vi "_sub_filter_raw_data.vi"(11 "raw data input":u32[](array[numeric])) -> (2 "Filtered raw data index":i32[](array[numeric]), 3 "Filtered raw data":u32[](array[numeric]))   [LabVIEW 2015]
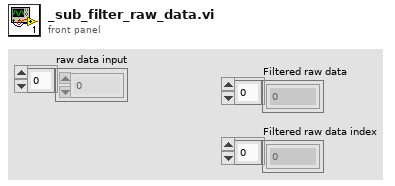
[diagram p1: front panel]
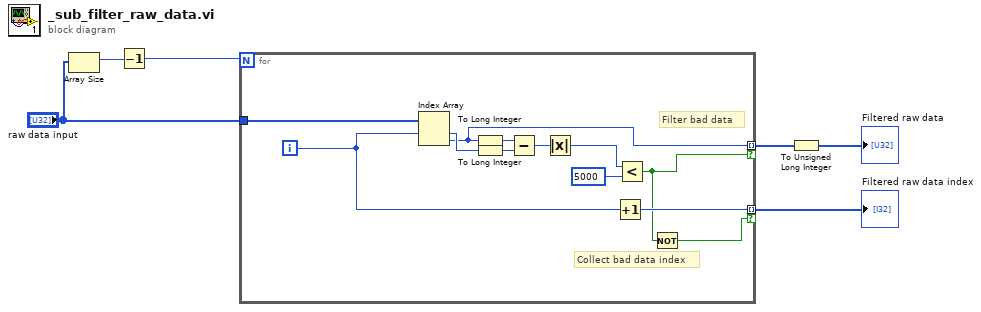
[diagram p0: block diagram]
diagram:
  n1 = Array Size(array="raw data input") -> (size(s)=w2:i32)
  n2 = Decrement(x=w2) -> (x-1=w1:i32)
  n3 = for {
    N: w1 -> [_]
    tunnel: "raw data input" -> [w18]
    tunnel: [w7] -> w6 mode=indexing if=w10
    tunnel: [w11] -> w5 mode=indexing if=w9
    i -> [w12]
    # "Collect bad data index"
    # "Filter bad data"
    n4 = Index Array(array=w18, index #1=w12) -> (element #1=w8:u32, element #2=w7:u32)  [unwired: 1 in]
    n5 = To Long Integer(number=w7) -> (32bit integer=w17:i32)
    n6 = To Long Integer(number=w8) -> (32bit integer=w16:i32)
    n7 = Subtract(x=w17, y=w16) -> (x-y=w15:i32)
    n8 = Absolute Value(x=w15) -> (abs(x)=w14:i32)
    n9 = Increment(x=w12) -> (x+1=w11:i32)
    n10 = Less?(x=w14, y=5000) -> (x < y?=w10:bool)
    n11 = Not(x=w10) -> (.not. x?=w9:bool)
  }
  "Filtered raw data index" <- w5
  n12 = To Unsigned Long Integer(number=w6) -> (unsigned 32bit integer=→"Filtered raw data":u32[])
